vi "SV TDMS Write XY (M Groups).vi"(0 "tdms file":refnum<k34>, 2 "write mode":u16(ring) items=["Append", "New group", "Overwrite"], 5 "group names in":string[](array[string]), 7 "channel name in":string="Channel0", 9 "XY":cluster{"X":dbl[], "Y":dbl[]}[](array[cluster]), 11 "error in":errorcluster, 12 "unit info":T5, 13 "function info":T4={"function type"=0, "function subtype"=2, "X-domain"=0} {"X-domain" items=["Time (s)"=0, "Frequency-CB (Hz)"=1, "Frequency-CPB (Hz)"=1248, "Frequency-Arbitrary (Hz)"=2357, "Quefrency (s)"=2, "Revolutions (rev)"=3, "Order"=4, "Speed (RPM)"=11, "Speed (rad/s)"=21, "Index"=65535]; "function subtype" items=["Unscaled binary"=0, "Scaled voltage"=1, "Scaled engineering units"=2, "-"=10, "Value"=19, "DC"=11, "AC"=12, "RMS^2"=13, "RMS"=14, "Peak"=15, "Peak to peak"=16, "-"=20, "1/1 octave"=21, "1/3 octave"=22, "1/6 octave"=23, "1/12 octave"=24, "1/24 octave"=25, "-"=30, "Density"=31, "Magnitude"=32, "Phase"=33, "Real"=34, "Imaginary"=35, "Complex"=345, "Coherence"=36, "-"=90, "Unknown"=99]; "function type" items=["Signal"=0, "Speed"=3, "Ratio"=6, "Count"=7, "-"=9, "Level"=10, "-"=19, "Octave Spectrum"=20, "-"=29, "FFT Auto Spectrum"=30, "FFT Cross Spectrum"=40, "Frequency Response"=50, "-"=59, "Event"=90]}) -> (4 "tdms file out":refnum<k34>, 6 "group names out":string[](array[string]), 15 "error out":errorcluster)   [LabVIEW 2017]
uses:
  <vilib>/addons/_NISVFA/_Shared subVIs/Controls/NI Function Type.ctl
  <vilib>/addons/_NISVFA/_Shared subVIs/Controls/NI Function SubType.ctl
  <vilib>/addons/_NISVFA/_Shared subVIs/Controls/svc_X-Axis Units.ctl
  <vilib>/addons/_NISVFA/_Shared subVIs/Controls/LV Datatypes.ctl
panel:
  out "channel name out":string
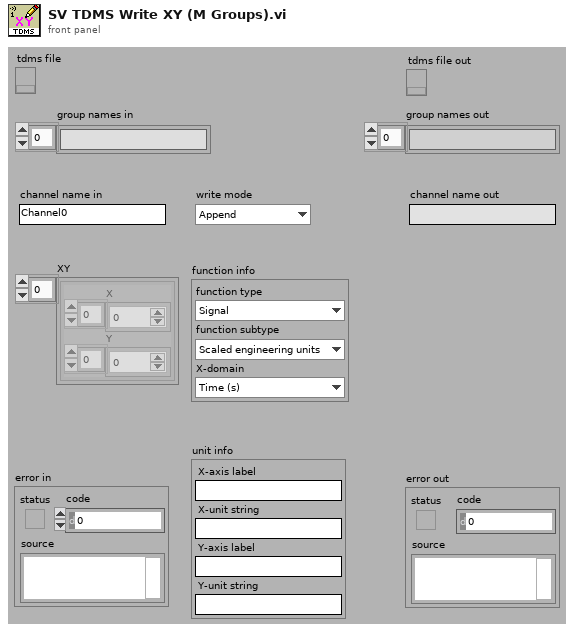
[diagram p1: front panel]
types:
  T1 = typedef "NI Function Type.ctl" = u16
  T2 = typedef "NI Function SubType.ctl" = u16
  T3 = typedef "svc_X-Axis Units.ctl" = u16
  T4 = cluster{"function type":T1, "function subtype":T2, "X-domain":T3}
  T5 = cluster{"X-axis label":string, "X-unit string":string, "Y-axis label":string, "Y-unit string":string}
  T6 = typedef "LV Datatypes.ctl" = i32
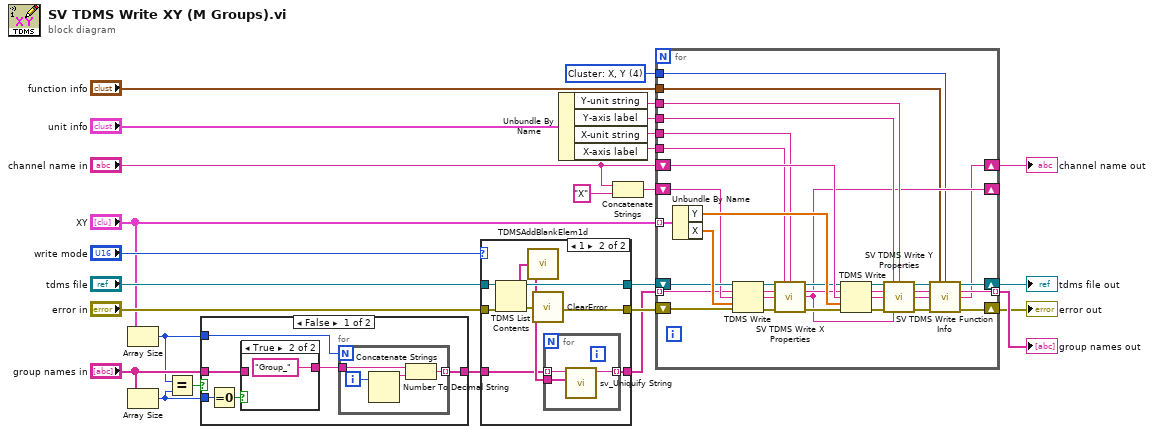
[diagram p0: block diagram]
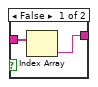
[diagram p2: hidden frame]
diagram:
  w1 = T6 4 items=["String: abc"=-2, "Boolean: True or False"=-1, "Scalar: y"=0, "Array: Y"=1, "Waveform: t0, dt, Y, variant"=2, "Cluster: x0, dx, Y"=3, "Cluster: X, Y"=4, "Waterfall"=5, "Colormap"=6] ("LabVIEW datatype")
  n1 = Array Size(array="XY") -> (size(s)=w9:i32)
  n2 = Array Size(array="group names in") -> (size(s)=w8:i32)
  n3 = Equal?(x=w9, y=w8) -> (x = y?=w11:bool)
  n4 = case shown="False" w11 {
    tunnel: "group names in" -> [w30 w40]
    tunnel: [w27 w40] -> w7
    tunnel: w8 -> [w32 _]
    tunnel: w9 -> [w29 _]
    frame False {
      n5 = Equal To 0?(x=w32) -> (x = 0?=w31:bool)
      n6 = case shown="True" w31 {
        tunnel: w30 -> [w38 _]
        tunnel: [w37 "Group_" ("channel name")] -> w28
        frame False {
          n7 = Index Array(array=w38) -> (element=w37:string)  [unwired: 1 in]
        }
        frame True {
        }
      }
      n8 = for {
        N: w29 -> [_]
        tunnel: w28 -> [w34]
        tunnel: [w33] -> w27 mode=indexing
        i -> [w35]
        n9 = Number To Decimal String(number=w35) -> (decimal integer string=w36:string)  [unwired: 1 in]
        n10 = Concatenate Strings(w34, w36) -> (w33:string)
      }
    }
    frame True {
    }
  }
  n11 = case shown="1" "write mode" {
    tunnel: [w43 w52] -> w18
    tunnel: [w41 w51] -> w16
    tunnel: w7 -> [w41 w46]
    tunnel: [w42 w49] -> w17
    tunnel: "error in" -> [w42 w48]
    tunnel: "tdms file" -> [w43 w47]
    frame 0, Default {
    }
    frame 1 {
      n12 = TDMS List Contents(4:w48, 7:w47) -> (0:w44:errorcluster, 2:w45:string[], 3:w52:refnum<k34>)  [unwired: 1 in, 1 out]
      n13 = call <vilib>:"TDMSAddBlankElem1d.vi"("input string array"=w45) -> ("output string array with blank element at the beginning"=w50:string[])
      n14 = call <vilib>:"ClearError.vi"("error in (no error)"=w44) -> ("error out"=w49:errorcluster)
      n15 = for {
        tunnel: [w55] -> w51 mode=indexing
        tunnel: w50 -> [w54]
        tunnel: w46 -> [w53] mode=indexing
        n16 = call <vilib>:"sv_Uniquify String.vi"("reserved strings"=w54, "string"=w53) -> ("unique string"=w55:string)  [unwired: 7 in, 2 out]
      }
    }
  }
  n17 = Unbundle By Name("unit info") -> ("Y-unit string"=w3:string, "Y-axis label"=w4:string, "X-unit string"=w5:string, "X-axis label"=w6:string)
  n18 = Concatenate Strings("channel name in", "X" ("string")) -> (w19:string)
  n19 = for {
    shift-right: [w61] -> w24
    shift-left: w18 -> [w85]
    shift-right: [w58] -> w21
    shift-left: w17 -> [w87]
    tunnel: "XY" -> [w89] mode=indexing
    tunnel: w16 -> [w82] mode=indexing
    tunnel: [w60] -> w23 mode=indexing
    shift-right: [w59] -> w13
    shift-left: "channel name in" -> [w84]
    shift-right: [w62] -> _
    shift-left: w19 -> [w83]
    tunnel: w6 -> [w77]
    tunnel: w5 -> [w76]
    tunnel: w4 -> [w72]
    tunnel: w3 -> [w71]
    tunnel: "function info" -> [w57]
    tunnel: w1 -> [w56]
    n20 = Unbundle By Name(w89) -> ("Y"=w88:dbl[], "X"=w86:dbl[])
    n21 = TDMS Write(0:w85, 5:w82, 7:w83, 9:w86, 11:w87) -> (4:w78:refnum<k34>, 6:w79:string, 8:w80:string, 15:w81:errorcluster)  [unwired: 1 in]
    n22 = call <vilib>:"SV TDMS Write X Properties.vi"("tdms file in"=w78, "X-axis label"=w77, "X-unit string"=w76, "group name"=w79, "channel name"=w80, "error in"=w81) -> ("tdms file out"=w74:refnum<k34>, "group name"=w73:string, "channel name"=w62:string, "error out"=w75:errorcluster)  [unwired: 6 in]
    n23 = TDMS Write(0:w74, 5:w73, 7:w84, 9:w88, 11:w75) -> (4:w70:refnum<k34>, 6:w69:string, 8:w68:string, 15:w67:errorcluster)  [unwired: 1 in]
    n24 = call <vilib>:"SV TDMS Write Y Properties.vi"("tdms file"=w70, "y-axis label"=w72, "y-unit string"=w71, "group name"=w69, "channel name"=w68, "error in (no error)"=w67, "xchannel name"=w62) -> ("tdms file out"=w63:refnum<k34>, "group name"=w64:string, "channel name"=w65:string, "error out"=w66:errorcluster)  [unwired: 5 in]
    n25 = call <vilib>:"SV TDMS Write Function Info.vi"("tdms file in"=w63, "function info"=w57, "LabVIEW datatype"=w56, "group name"=w64, "channel name"=w65, "error in (no error)"=w66) -> ("tdms file out"=w61:refnum<k34>, "group name out"=w60:string, "channel name out"=w59:string, "error out"=w58:errorcluster)  [unwired: 6 in]
  }
  "error out" <- w21
  "tdms file out" <- w24
  "group names out" <- w23
  "channel name out" <- w13
